vi "XIPIN_3GPP2_Turbo_Decoder_2_1.vi"   [LabVIEW 2017]
doc: "Rev 1. The 3GPP2 Turbo Decoder from Xilinx is a high-speed, compact core which offers support for specifications, '3GPP2 C.S0024-A V2.0' and '3GPP2 C.S0024-B V1.0'. The Turbo Decoder core is parameterizable allowing the designer to trade-off Bit Error Rate (BER) against core complexity and performance. The core is delivered through the Xilinx CORE Generator System and integrates seamlessly with the Xilinx design flow.\n------------------------------------\n<b>Need License</b> : Yes"
uses:
  <vilib>/rvi/XilinxIP/XIPIN_XNode/niFpgaXIPIN.xnode
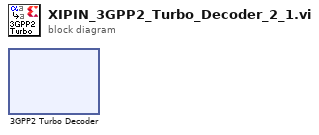
[diagram p0: block diagram]
diagram:
  n1 = xnode ("3GPP2 Turbo Decoder")() -> ()
